vi "Closing_Sessions.vi"(0 "DCPowerInformationClusterArray_Input":T2(array[cluster]), 1 "Oscilloscope Configuration Input Array":T5(array[cluster]) {"vertical coupling" items=["AC", "DC", "Ground"]}, 2 "error in (no error)":errorcluster, 3 "RF Block Input Array":T3[](array[typedef]), 4 "VISAPowerInfoInputArray":T1[](array[typedef])) -> (5 "Oscilloscope Configuration Output Array":T5(array[cluster]) {"vertical coupling" items=["AC", "DC", "Ground"]}, 6 "DCPowerInformationClusterArray_Output":T2(array[cluster]), 7 "error out":errorcluster, 8 "VISAPowerInfo Output Array":T1[](array[typedef]), 9 "RF Block Output Array":T3[](array[typedef]))   [LabVIEW 2019]
uses:
  <instrlib>/niScope/Controls/niScope vertical coupling.ctl
  Controls/RFBlockControl.ctl
  Controls/VISA_power_Control.ctl
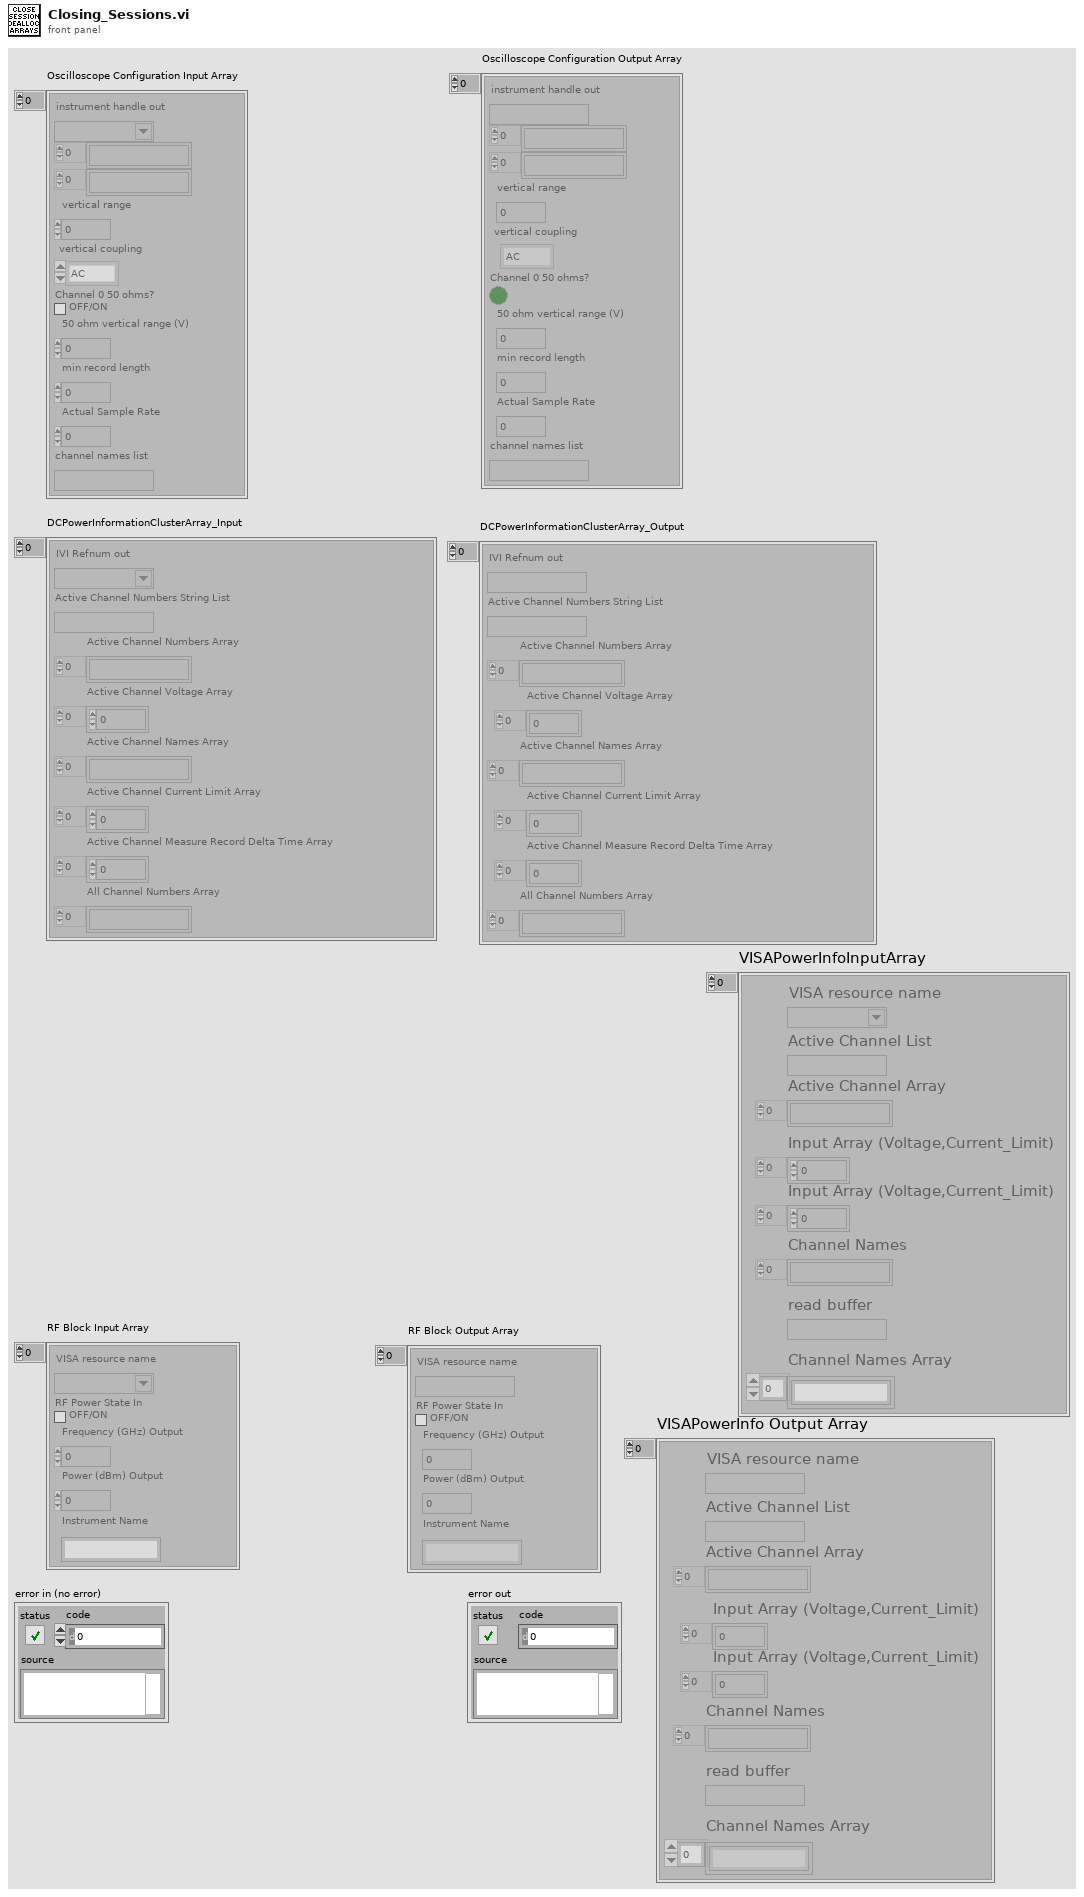
[diagram p1: front panel]
types:
  T1 = typedef "VISA_power_Control.ctl" = cluster{"VISA resource name":refnum<visa-resource-name>, "Active Channel List":string, "Active Channel Array":string[], "Input Array (Voltage,Current_Limit)":dbl[], "Input Array (Voltage,Current_Limit)":dbl[], "Channel Names":string[], "read buffer":string, "Channel Names Array":string[]}
  T2 = cluster{"IVI Refnum out":refnum<k15>, "Active Channel Numbers String List":string, "Active Channel Numbers Array":string[], "Active Channel Voltage Array":dbl[], "Active Channel Names Array":string[], "Active Channel Current Limit Array":dbl[], "Active Channel Measure Record Delta Time Array":dbl[], "All Channel Numbers Array":string[]}[]
  T3 = typedef "RFBlockControl.ctl" = cluster{"VISA resource name":refnum<visa-resource-name>, "RF Power State In":bool, "Frequency (GHz) Output":dbl, "Power (dBm) Output":dbl, "Instrument Name":string}
  T4 = typedef "niScope vertical coupling.ctl" = i32
  T5 = cluster{"instrument handle out":refnum<k15>, string[], string[], "vertical range":dbl, "vertical coupling":T4, "Channel 0 50 ohms?":bool, "50 ohm vertical range (V)":dbl, "min record length":i32, "Actual Sample Rate":dbl, "channel names list":string}[]
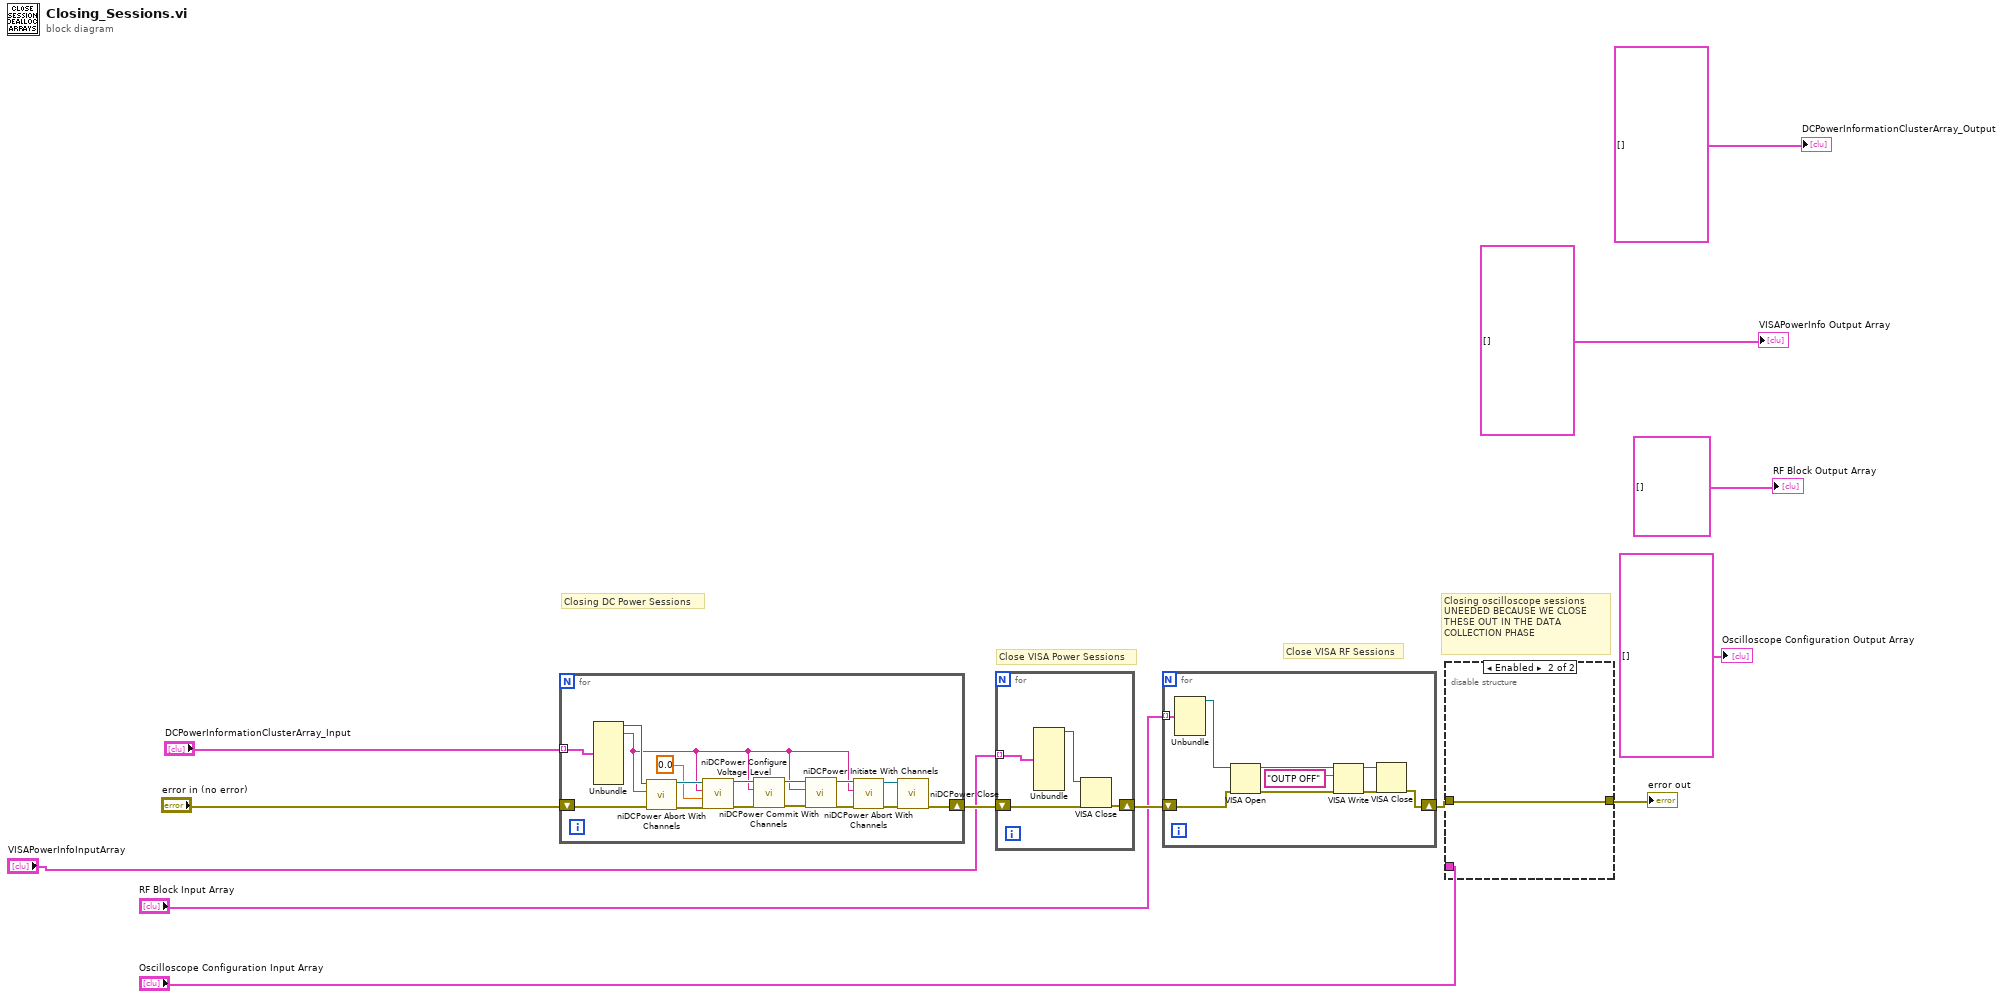
[diagram p0: block diagram]
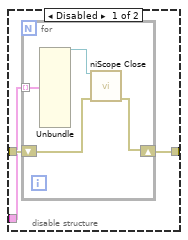
[diagram p2: hidden frame]
diagram:
  # "Closing oscilloscope sessions \nUNEEDED BECAUSE WE CLOSE THESE OUT IN THE DATA COLLECTION PHASE"
  # "Close VISA RF Sessions"
  # "Close VISA Power Sessions"
  # "Closing DC Power Sessions"
  n1 = for {
    tunnel: "DCPowerInformationClusterArray_Input" -> [w29] mode=indexing
    shift-right: [w28] -> w8
    shift-left: "error in (no error)" -> [w24]
    n2 = Unbundle(w29) -> ("IVI Refnum out"=w25:refnum<k15>, "Active Channel Numbers String List"=w14:string)  [unwired: 6 out]
    n3 = call <instrlib>:"niDCPower Abort With Channels.vi"("error in (no error)"=w24, "channel name"=w14, "instrument handle"=w25) -> ("error out"=w27:errorcluster, "instrument handle out"=w26:refnum<k15>)  [unwired: 7 in]
    n4 = call <instrlib>:"niDCPower Configure Voltage Level.vi"("error in (no error)"=w27, "voltage level"=0.0, "channel name"=w14, "instrument handle"=w26) -> ("error out"=w19:errorcluster, "instrument handle out"=w20:refnum<k15>)  [unwired: 6 in]
    n5 = call <instrlib>:"niDCPower Commit With Channels.vi"("error in (no error)"=w19, "channel name"=w14, "instrument handle"=w20) -> ("error out"=w21:errorcluster, "instrument handle out"=w22:refnum<k15>)  [unwired: 7 in]
    n6 = call <instrlib>:"niDCPower Initiate With Channels.vi"("error in (no error)"=w21, "channel name"=w14, "instrument handle"=w22) -> ("error out"=w16:errorcluster, "instrument handle out"=w15:refnum<k15>)  [unwired: 7 in]
    n7 = call <instrlib>:"niDCPower Abort With Channels.vi"("error in (no error)"=w16, "channel name"=w14, "instrument handle"=w15) -> ("error out"=w18:errorcluster, "instrument handle out"=w17:refnum<k15>)  [unwired: 7 in]
    n8 = call <instrlib>:"niDCPower Close.vi"("error in (no error)"=w18, "instrument handle"=w17) -> ("error out"=w28:errorcluster)  [unwired: 9 in]
  }
  n9 = for {
    tunnel: "VISAPowerInfoInputArray" -> [w33] mode=indexing
    shift-right: [w30] -> w10
    shift-left: w8 -> [w31]
    n10 = Unbundle(w33) -> ("VISA resource name"=w32:refnum<visa-resource-name>)  [unwired: 7 out]
    n11 = VISA Close(VISA resource name=w32, error in (no error)=w31) -> (error out=w30:errorcluster)
  }
  n12 = for {
    tunnel: "RF Block Input Array" -> [w42] mode=indexing
    shift-right: [w41] -> w12
    shift-left: w10 -> [w34]
    n13 = Unbundle(w42) -> ("VISA resource name"=w36:refnum<visa-resource-name>)  [unwired: 4 out]
    n14 = VISA Open(error in (no error)=w34, VISA resource name=w36) -> (VISA resource name=w35:refnum<visa-resource-name>, error out=w37:errorcluster)  [unwired: 3 in]
    n15 = VISA Write(VISA resource name=w35, write buffer="OUTP OFF", error in (no error)=w37) -> (VISA resource name out=w39:refnum<visa-resource-name>, error out=w40:errorcluster)  [unwired: 1 out]
    n16 = VISA Close(VISA resource name=w39, error in (no error)=w40) -> (error out=w41:errorcluster)
  }
  n17 = disable-structure shown="Enabled" {
    disable-tunnel: [w45 w50] -> w13
    disable-tunnel: w12 -> [w44 w50]
    disable-tunnel: "Oscilloscope Configuration Input Array" -> [w43 _]
    frame Disabled {
      n18 = for {
        tunnel: w43 -> [w49] mode=indexing
        shift-right: [w47] -> w45
        shift-left: w44 -> [w48]
        n19 = Unbundle(w49) -> ("instrument handle out"=w46:refnum<k15>)  [unwired: 9 out]
        n20 = call <instrlib>:"niScope Close.vi"("instrument handle"=w46, "error in"=w48) -> ("error out"=w47:errorcluster)  [unwired: 13 in]
      }
    }
    frame Enabled {
    }
  }
  "error out" <- w13
  "Oscilloscope Configuration Output Array" <- T5 [] ("Oscilloscope Configuration Input Array")
  "RF Block Output Array" <- T3[] [] ("RF Block Input Array")
  "DCPowerInformationClusterArray_Output" <- T2 [] ("DCPowerInformationClusterArray_Input")
  "VISAPowerInfo Output Array" <- T1[] [] ("VISAPowerInfoInputArray")
